vi "Close Queues.vi"(7 "QRD":T1, 8 "error in":errorcluster) -> (0 "error out":errorcluster, 5 "QRD Out":T1)   [LabVIEW 2025]
uses:
  Controls/Queues-Refs-Data.ctl
  Builds/Queue Wrappers.lvlibp/Q Packet.ctl
  Builds/Queue Wrappers.lvlibp
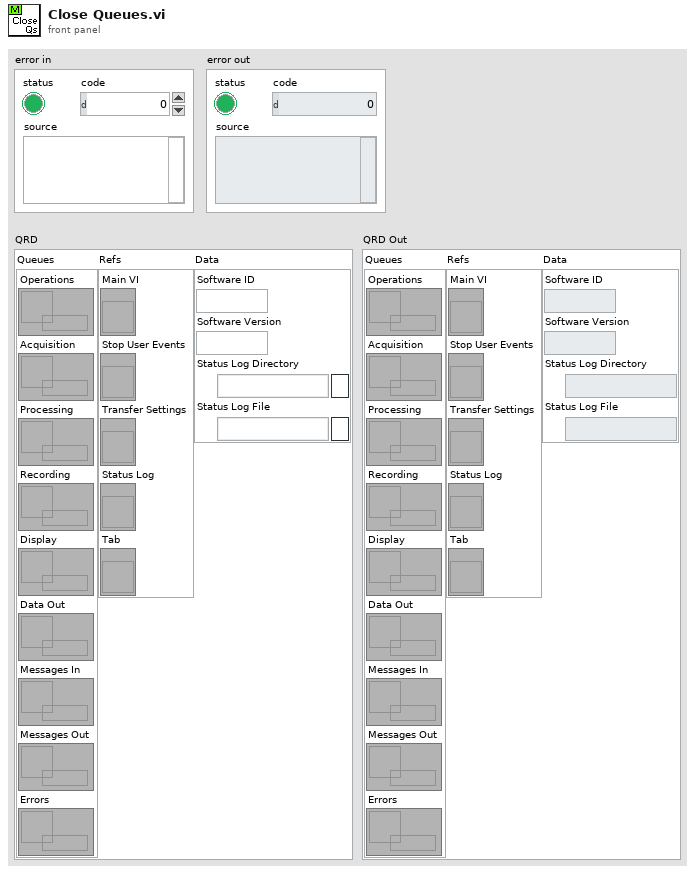
[diagram p1: front panel]
types:
  T1 = typedef "Queues-Refs-Data.ctl" = cluster{"Queues":cluster{"Operations":refnum<queue>, "Acquisition":refnum<queue>, "Processing":refnum<queue>, "Recording":refnum<queue>, "Display":refnum<queue>, "Data Out":refnum<queue>, "Messages In":refnum<queue>, "Messages Out":refnum<queue>, "Errors":refnum<queue>}, "Refs":cluster{"Main VI":refnum<vi>, "Stop User Events":refnum<vi>, "Transfer Settings":refnum<vi>, "Status Log":refnum<vi>, "Tab":refnum<vi>}, "Data":cluster{"Software ID":string, "Software Version":string, "Status Log Directory":path, "Status Log File":path}}
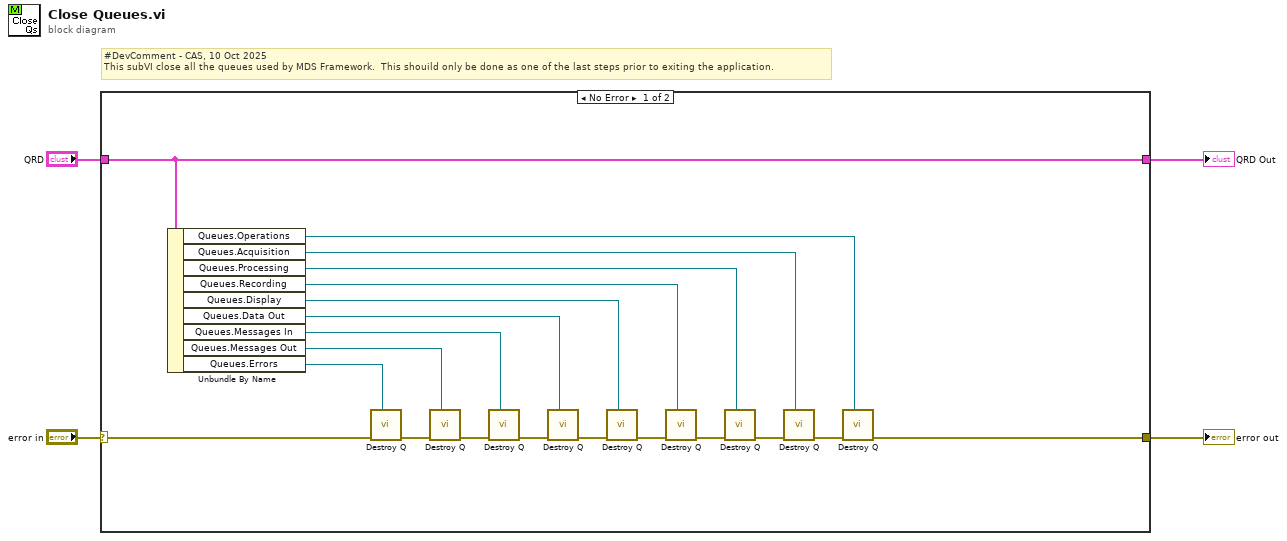
[diagram p0: block diagram]
diagram:
  # "#DevComment - CAS, 10 Oct 2025\nThis subVI close all the queues used by MDS Framework.  This shouild only be done as one of the last steps prior to exiting the application."
  n1 = case shown="No Error" "error in" {
    selector: "error in" -> [w22 w26]
    tunnel: "QRD" -> [w24 w25]
    tunnel: [w5 w26] -> w2
    tunnel: [w24 w25] -> w1
    frame No Error {
      n2 = Unbundle By Name(w24) -> ("Queues.Operations"=w6:refnum<queue>, "Queues.Acquisition"=w8:refnum<queue>, "Queues.Processing"=w9:refnum<queue>, "Queues.Recording"=w10:refnum<queue>, "Queues.Display"=w11:refnum<queue>, "Queues.Data Out"=w12:refnum<queue>, "Queues.Messages In"=w13:refnum<queue>, "Queues.Messages Out"=w14:refnum<queue>, "Queues.Errors"=w23:refnum<queue>)
      n3 = call "Destroy Q.vi"("Q Ref In"=w23, "error in"=w22) -> ("error out"=w21:errorcluster)  [unwired: 8 in, 1 out]
      n4 = call "Destroy Q.vi"("Q Ref In"=w14, "error in"=w21) -> ("error out"=w19:errorcluster)  [unwired: 8 in, 1 out]
      n5 = call "Destroy Q.vi"("Q Ref In"=w13, "error in"=w19) -> ("error out"=w20:errorcluster)  [unwired: 8 in, 1 out]
      n6 = call "Destroy Q.vi"("Q Ref In"=w12, "error in"=w20) -> ("error out"=w15:errorcluster)  [unwired: 8 in, 1 out]
      n7 = call "Destroy Q.vi"("Q Ref In"=w11, "error in"=w15) -> ("error out"=w16:errorcluster)  [unwired: 8 in, 1 out]
      n8 = call "Destroy Q.vi"("Q Ref In"=w10, "error in"=w16) -> ("error out"=w18:errorcluster)  [unwired: 8 in, 1 out]
      n9 = call "Destroy Q.vi"("Q Ref In"=w9, "error in"=w18) -> ("error out"=w17:errorcluster)  [unwired: 8 in, 1 out]
      n10 = call "Destroy Q.vi"("Q Ref In"=w8, "error in"=w17) -> ("error out"=w7:errorcluster)  [unwired: 8 in, 1 out]
      n11 = call "Destroy Q.vi"("Q Ref In"=w6, "error in"=w7) -> ("error out"=w5:errorcluster)  [unwired: 8 in, 1 out]
    }
    frame Error {
    }
  }
  "error out" <- w2
  "QRD Out" <- w1
